vi "load_channel_settings.vi"(8 "error in":errorcluster) -> (0 "error out":errorcluster, 3 "swabian_channel_settings":T1=[{"Threshold (V)"=0.5, "Input Delay (ps)"=0, "Dead Time (ps)"=6000}, {"Threshold (V)"=0.5, "Input Delay (ps)"=0, "Dead Time (ps)"=6000}, {"Threshold (V)"=0.5, "Input Delay (ps)"=0, "Dead Time (ps)"=6000}, {"Threshold (V)"=0.5, "Input Delay (ps)"=0, "Dead Time (ps)"=6000}, {"Threshold (V)"=0.5, "Input Delay (ps)"=0, "Dead Time (ps)"=6000}, {"Threshold (V)"=0.5, "Input Delay (ps)"=0, "Dead Time (ps)"=6000}, {"Threshold (V)"=0.5, "Input Delay (ps)"=0, "Dead Time (ps)"=6000}, {"Threshold (V)"=0.5, "Input Delay (ps)"=0, "Dead Time (ps)"=6000}] {"Dead Time (ps)" min=0 step=6000; "Input Delay (ps)" min=0 step=1; "Threshold (V)" min=0.0 max=2.5 step=0.1})   [LabVIEW 2018]
uses:
  swabian_channel_settings.ctl
  channel_settings.ctl
  <vilib>/Utility/xml.llb/Read From XML File(string).vi
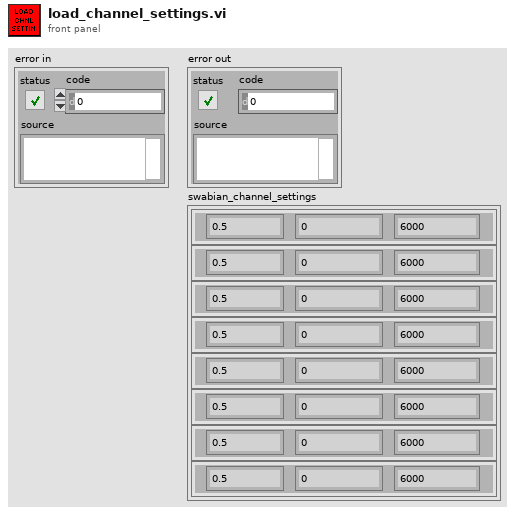
[diagram p1: front panel]
types:
  T1 = typedef "swabian_channel_settings.ctl" = T2[]
  T2 = typedef "channel_settings.ctl" = cluster{"Threshold (V)":dbl, "Input Delay (ps)":i64, "Dead Time (ps)":i64}
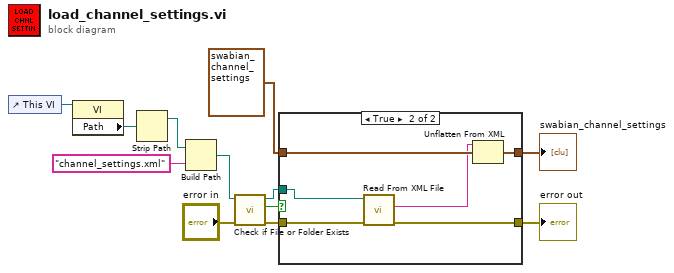
[diagram p0: block diagram]
diagram:
  n1 = control-ref of="This VI"() -> (w12:refnum<vi>)
  n2 = property class="VI"(reference=w12) -> ("Path"=w11:path)  [unwired: 1 in, 2 out]
  n3 = Strip Path(path=w11) -> (stripped path=w10:path)  [unwired: 1 out]
  n4 = Build Path(base path=w10, name or relative path="channel_settings.xml") -> (appended path=w7:path)
  n5 = call <vilib>:"Check if File or Folder Exists.vi"("error in (no error)"="error in", "path"=w7) -> ("error out"=w5:errorcluster, "file or folder exists?"=w4:bool, "dup path"=w1:path)  [unwired: 7 in]
  n6 = case shown="True" w4 {
    tunnel: w5 -> [w14 w18]
    tunnel: [w14 w15] -> w8
    tunnel: T1 [{"Threshold (V)"=0.5, "Input Delay (ps)"=0, "Dead Time (ps)"=6000}, {"Threshold (V)"=0.5, "Input Delay (ps)"=0, "Dead Time (ps)"=6000}, {"Threshold (V)"=0.5, "Input Delay (ps)"=0, "Dead Time (ps)"=6000}, {"Threshold (V)"=0.5, "Input Delay (ps)"=0, "Dead Time (ps)"=6000}, {"Threshold (V)"=0.5, "Input Delay (ps)"=0, "Dead Time (ps)"=6000}, {"Threshold (V)"=0.5, "Input Delay (ps)"=0, "Dead Time (ps)"=6000}, {"Threshold (V)"=0.5, "Input Delay (ps)"=0, "Dead Time (ps)"=6000}, {"Threshold (V)"=0.5, "Input Delay (ps)"=0, "Dead Time (ps)"=6000}] ("swabian_channel_settings") -> [w13 w20]
    tunnel: [w13 w19] -> w2
    tunnel: w1 -> [_ w17]
    frame False {
    }
    frame True {
      n7 = call-poly <vilib>:"Read From XML File.vi"("error in (no error)"=w18, "XML File Path"=w17) -> ("error out"=w15:errorcluster, "XML Elements"=w16:string)  [unwired: 7 in, 1 out]
      n8 = Unflatten From XML(xml string=w16, type=w20) -> (value=w19:T1)  [unwired: 1 in, 1 out]
    }
  }
  "error out" <- w8
  "swabian_channel_settings" <- w2
